vi "Output interface.vi"(6 "Stamp Command":T6, 8 "error in":errorcluster, 10 "Control":T1 {"Pumps"."0 to 1" format="%.2f"; "Pumps"."flow rate" format="%.2f"}, 11 "DeviceName":string) -> (0 "error out":errorcluster, 1 "success?":bool)   [LabVIEW 2019]
uses:
  Stamp/stamp command.ctl
  Stamp/Stamp 2 control.ctl
  Peristaltic/Pump w direction.ctl
  Stamp/mini peristaltic pump.ctl
  Stamp/Pump Direction.ctl
  Stamp/3-stop colors and numbers.ctl
  <vilib>/DAQmx/write.llb/DAQmx Write (Analog 1D DBL NChan 1Samp).vi
  <vilib>/DAQmx/write.llb/DAQmx Write (Digital 2D Bool NChan 1Samp NLine).vi
  <vilib>/DAQmx/create/channels.llb/DAQmx Create Channel (AO-Voltage-Basic).vi
  <vilib>/DAQmx/create/channels.llb/DAQmx Create Channel (DO-Digital Output).vi
  <vilib>/DAQmx/miscellaneous.llb/DAQmx Fill In Error Info.vi
panel:
  out "error out 2":errorcluster
  out "Pump volts":dbl[](array[numeric])
  out "sending to DO":bool[][](array[boolean])
  out "AO":string
  out "DO":string
  # "0-12"
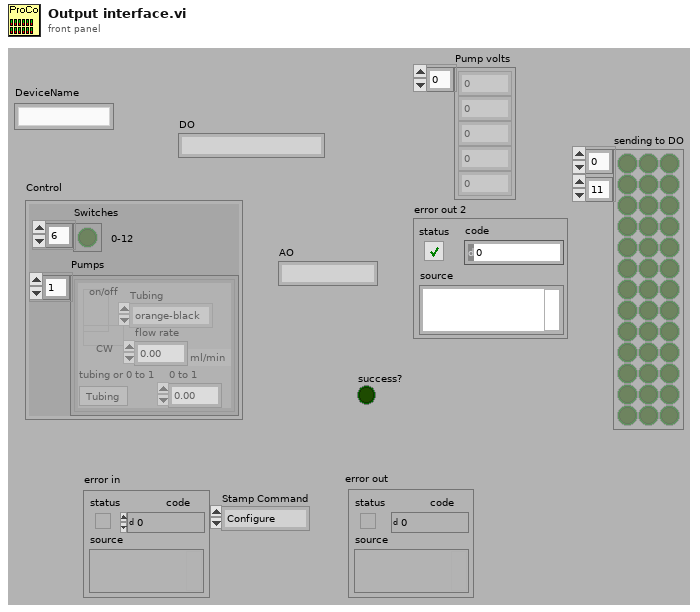
[diagram p1: front panel]
types:
  T1 = typedef "Stamp 2 control.ctl" = cluster{"Switches":bool[], "Pumps":T2[]}
  T2 = typedef "Pump w direction.ctl" = cluster{"on/off":T3, "Direction":T4, "flow rate":dbl[unit], "Tubing":T5, "tubing or 0 to 1":bool, "0 to 1":dbl}
  T3 = typedef "mini peristaltic pump.ctl" = bool
  T4 = typedef "Pump Direction.ctl" = bool
  T5 = typedef "3-stop colors and numbers.ctl" = enum16{"orange-black", "orange-red", "orange-blue", "orange-green", "green-yellow", "orange-yellow", "white-yellow", "orange-white", "black-black", "orange-orange", "white-black", "white-white", "white-red", "red-red", "red-grey", "grey-grey", "yellow-yellow", "yellow-blue", "blue-blue", "blue-green", "green-green", "purple-purple", "purple-black", "purple-orange", "purple-white", "black-white", "13", "14", "15", "16", "17", "18"}
  T6 = typedef "stamp command.ctl" = enum16{"Configure", "Write", "Off", "Close"}
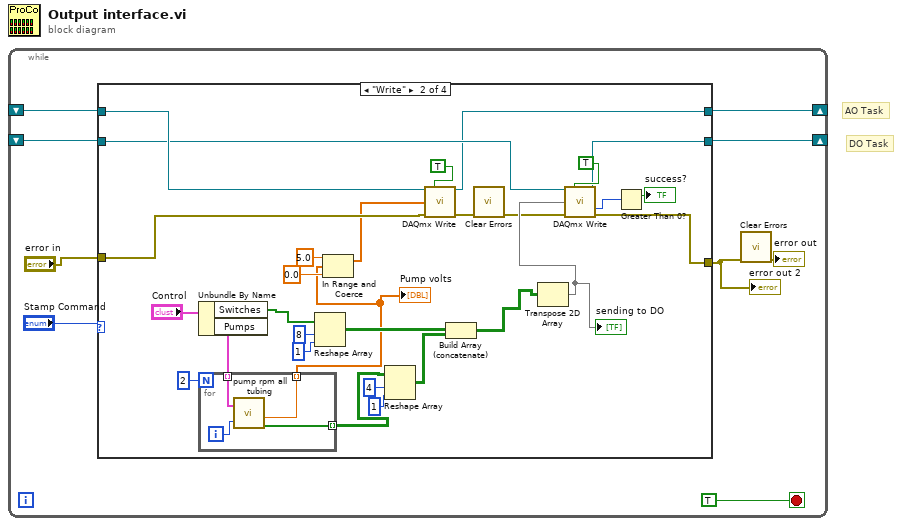
[diagram p0: block diagram]
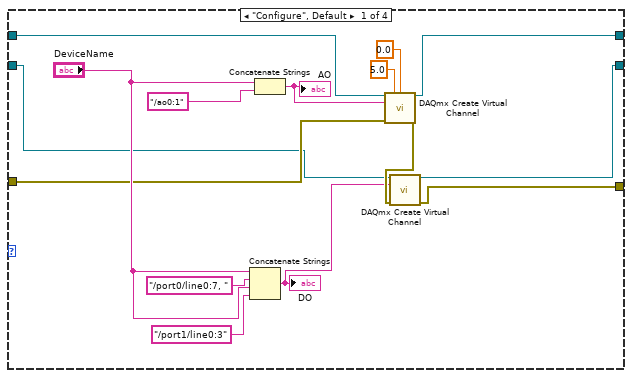
[diagram p2: hidden frame]
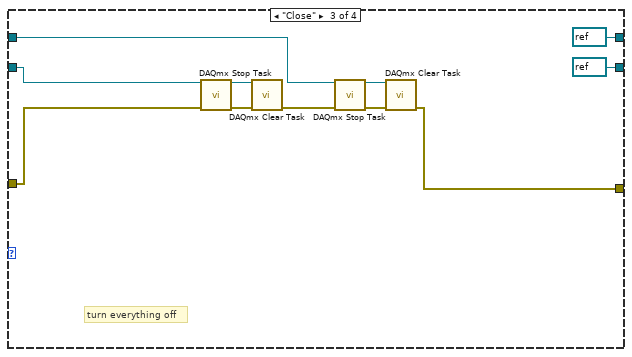
[diagram p3: hidden frame]
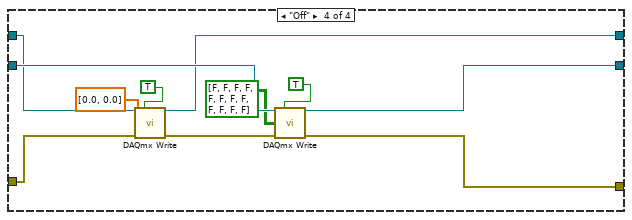
[diagram p4: hidden frame]
diagram:
  # "DO Task"
  # "AO Task"
  n1 = while {
    shift-right: [w5] -> _
    shift-left: _ -> [w3]
    shift-right: [w4] -> _
    shift-left: _ -> [w2]
    stop <- TRUE stop-if-true
    n2 = case shown="\"Write\"" "Stamp Command" {
      tunnel: "error in" -> [w16 w46 w66 w73]
      tunnel: [w14 w35 w60 w71] -> w6
      tunnel: [w18 w42 refnum<k21> refnum ("task out") w74] -> w5
      tunnel: [w17 w43 refnum<k21> refnum ("task out") w76] -> w4
      tunnel: w3 -> [w11 w45 w64 w75]
      tunnel: w2 -> [w10 w44 w65 w77]
      frame "Configure", Default {
        n3 = Concatenate Strings("DeviceName", "/port0/line0:7, ", "DeviceName", "/port1/line0:3") -> (w12:string)
        "DO" <- w12
        n4 = Concatenate Strings("DeviceName", "/ao0:1") -> (w13:string)
        "AO" <- w13
        n5 = call-poly <vilib>:"DAQmx Create Virtual Channel.vi"("task in"=w11, "maximum value"=5.0, "minimum value"=0.0, "physical channels"=w13, "error in"=w16) -> ("task out"=w18:refnum<k21>, "error out"=w15:errorcluster)  [unwired: 9 in]
        n6 = call-poly <vilib>:"DAQmx Create Virtual Channel.vi"("task in"=w10, "lines"=w12, "error in"=w15) -> ("task out"=w17:refnum<k21>, "error out"=w14:errorcluster)  [unwired: 11 in]
      }
      frame "Write" {
        n7 = Unbundle By Name("Control") -> ("Switches"=w51:bool[], "Pumps"=w52:T2[])
        n8 = for {
          N: 2 -> [_]
          tunnel: w52 -> [w57] mode=indexing
          tunnel: [w55] -> w39 mode=indexing
          tunnel: [w54] -> w26 mode=indexing
          i -> [w56]
          n9 = call "pump rpm all tubing.vi"("Pump"=w57, "pump ID"=w56) -> ("pump volts (0-5)"=w54:dbl, "Pump dir on"=w55:T3[])  [unwired: 1 in, 1 out]
        }
        "Pump volts" <- w26
        n10 = Reshape Array(w51, 8 ("dimension size"), 1 ("dimension size")) -> (w41:bool[][])
        n11 = In Range and Coerce(upper limit=5.0, x=w26, lower limit=0.0) -> (coerced(x)=w25:dbl[])  [unwired: 1 out]
        n12 = Reshape Array(w39, 4 ("dimension size"), 1 ("dimension size")) -> (w38:T3[][])
        n13 = call-poly <vilib>:"DAQmx Write.vi"("task/channels in"=w45, "auto start"=TRUE, "data"=w25, "error in"=w46) -> ("task out"=w42:refnum<k21>, "error out"=w47:errorcluster)  [unwired: 9 in, 1 out]
        n14 = Build Array (concatenate)(w41, w38) -> (w31:T3[][])
        n15 = call <vilib>:"Clear Errors.vi"("error in (no error)"=w47) -> ("error out"=w29:errorcluster)  [unwired: 5 in, 1 out]
        n16 = Transpose 2D Array(2D array=w31) -> (transposed array=w30:T3[][])
        "sending to DO" <- w30
        n17 = call-poly <vilib>:"DAQmx Write.vi"("task/channels in"=w44, "auto start"=TRUE, "data"=w30, "error in"=w29) -> ("task out"=w43:refnum<k21>, "number of samples written per channel"=w34:u32, "error out"=w35:errorcluster)  [unwired: 9 in]
        n18 = Greater Than 0?(x=w34) -> (x > 0?=→"success?":bool)
      }
      frame "Close" {
        # "turn everything off"
        n19 = call <vilib>:"DAQmx Stop Task.vi"("task/channels in"=w65, "error in"=w66) -> ("task out"=w67:refnum<k21>, "error out"=w68:errorcluster)  [unwired: 12 in]
        n20 = call <vilib>:"DAQmx Clear Task.vi"("task in"=w67, "error in"=w68) -> ("error out"=w63:errorcluster)  [unwired: 13 in]
        n21 = call <vilib>:"DAQmx Stop Task.vi"("task/channels in"=w64, "error in"=w63) -> ("task out"=w61:refnum<k21>, "error out"=w62:errorcluster)  [unwired: 12 in]
        n22 = call <vilib>:"DAQmx Clear Task.vi"("task in"=w61, "error in"=w62) -> ("error out"=w60:errorcluster)  [unwired: 13 in]
      }
      frame "Off" {
        n23 = call-poly <vilib>:"DAQmx Write.vi"("task/channels in"=w75, "auto start"=TRUE, "data"=dbl[] [0.0, 0.0], "error in"=w73) -> ("task out"=w74:refnum<k21>, "error out"=w72:errorcluster)  [unwired: 9 in, 1 out]
        n24 = call-poly <vilib>:"DAQmx Write.vi"("task/channels in"=w77, "auto start"=TRUE, "data"=bool[][] [[FALSE, FALSE, FALSE, FALSE, FALSE, FALSE, FALSE, FALSE, FALSE, FALSE, FALSE, FALSE]], "error in"=w72) -> ("task out"=w76:refnum<k21>, "error out"=w71:errorcluster)  [unwired: 9 in, 1 out]
      }
    }
    "error out 2" <- w6
    n25 = call <vilib>:"Clear Errors.vi"("error in (no error)"=w6) -> ("error out"=→"error out":errorcluster)  [unwired: 5 in, 1 out]
  }
